vi "stat_f_s1.vi"(6 "kD":dbl=1.3, 7 "Y":dbl[](array[numeric])) -> (1 "stops":i32[](array[numeric]), 2 "starts":i32[](array[numeric]), 3 "mean":dbl format="%0.2f")   [LabVIEW 2010]
uses:
  <vilib>/Analysis/NI_AALBase.lvlib
panel:
  out "Array":i32[](array[numeric])
  out "Waveform Graph":cluster{"Numeric":i32, i32, dbl[]}(graph)
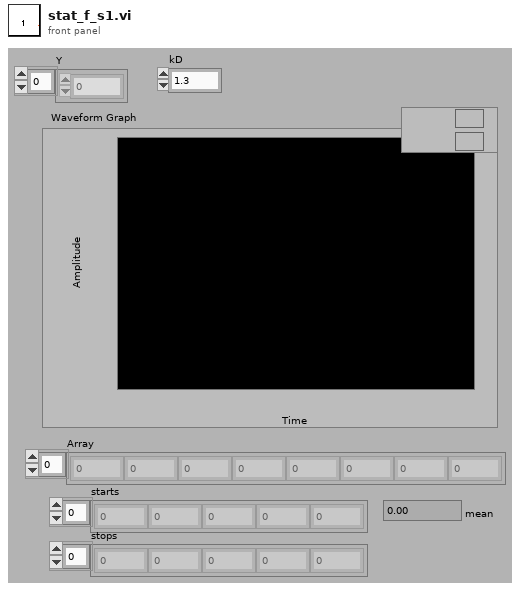
[diagram p1: front panel]
types:
  T1 = cluster{"Name":string, "Color":u32, "Style":u8, "Point Style":u8, "Name Visible":bool, "Allow Drag":bool, "Lock Style":u32, "Plot":u32, "Index":i32, "Position":cluster{"X":dbl, "Y":dbl}}[]
  T2 = cluster{"Name":string, "Color":u32, "Style":u8, "Point Style":u8, "Name Visible":bool, "Allow Drag":bool, "Lock Style":u32, "Plot":u32, "Index":i32, "Position":cluster{"X":dbl, "Y":dbl}}
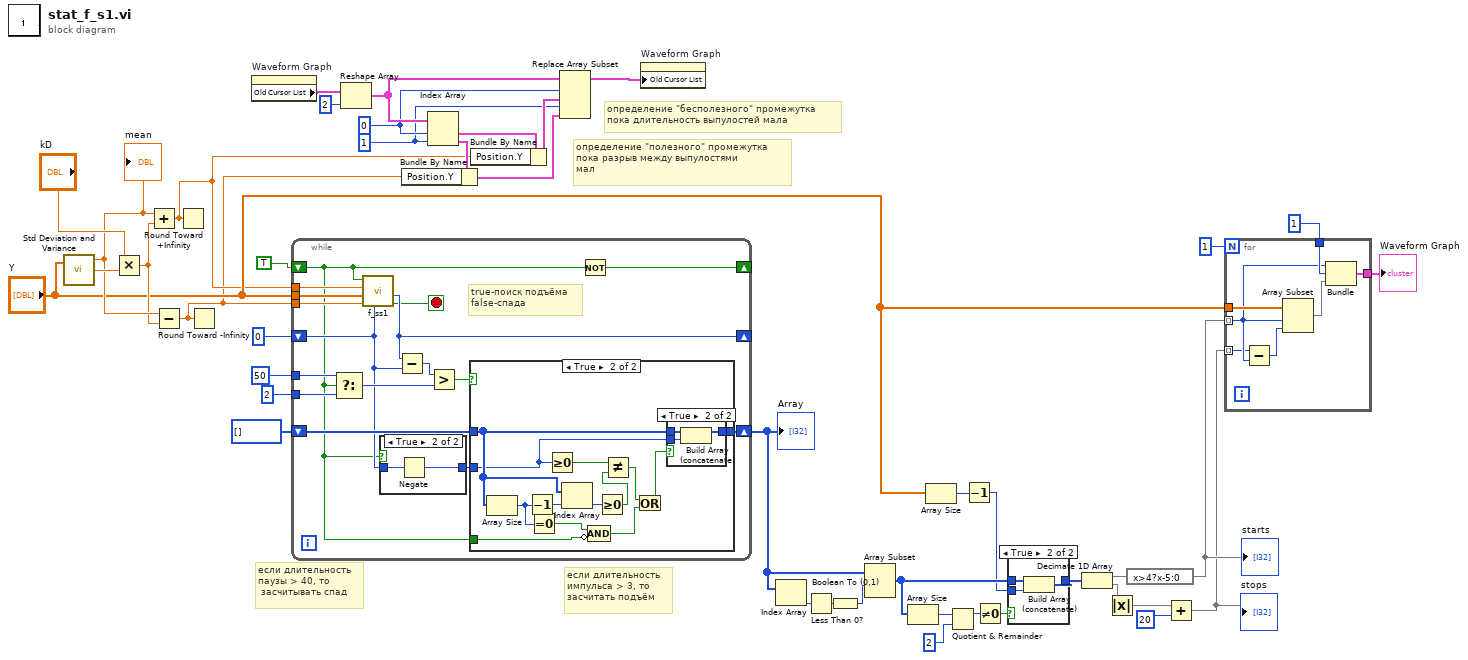
[diagram p0: block diagram]
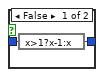
[diagram p3: hidden frame]
diagram:
  w34 = 1 ("index")
  w35 = 0 ("index")
  # "если длительность\nимпульса > 3, то\nзасчитать подъём"
  # "если длительность\nпаузы > 40, то\n засчитывать спад"
  # "определение \"полезного\" промежутка\nпока разрыв между выпулостями\nмал"
  # "определение \"бесполезного\" промежутка\nпока длительность выпулостей мала"
  n1 = call <vilib>:"Std Deviation and Variance.vi"("X"="Y") -> ("mean"=w27:dbl, "standard deviation"=w28:dbl)  [unwired: 1 in, 1 out]
  "mean" <- w27
  n2 = Multiply(x="kD", y=w28) -> (x*y=w26:dbl)
  n3 = Add(x=w27, y=w26) -> (x+y=w2:dbl)
  n4 = Subtract(x=w27, y=w26) -> (x-y=w1:dbl)
  n5 = Round Toward +Infinity(x=w2) -> ()  [unwired: 1 out]
  n6 = Round Toward -Infinity(1:w1) -> ()  [unwired: 1 out]
  n7 = property on="Waveform Graph" class="WFGraph (strict)"() -> ("Old Cursor List"=w43:T1)  [unwired: 2 in, 2 out]
  n8 = while {
    tunnel: w1 -> [w56]
    tunnel: w2 -> [w57]
    tunnel: "Y" -> [w58]
    shift-right: [w54] -> _
    shift-left: 0 -> [w46]
    shift-right: [w55] -> _
    shift-left: TRUE ("Boolean") -> [w44]
    tunnel: 50 ("t") -> [w51]
    tunnel: 2 -> [w50]
    shift-right: [w48] -> w20
    shift-left: i32[] [] -> [w47]
    stop <- w53 stop-if-true
    # "true-поиск подъёма\nfalse-спада"
    n9 = Select(t=w51, s=w44, f=w50) -> (s? t:f=w49:i32)
    n10 = call "f_ss1.vi"("index in"=w46, "lower lim"=w56, "Y"=w58, "upper lim"=w57, "Boolean"=w44) -> ("eof"=w53:bool, "index out"=w54:i32)  [unwired: 1 in, 1 out]
    n11 = case shown="True" w44 {
      tunnel: [w61 w62] -> w45
      tunnel: w46 -> [w60 w63]
      frame False {
        n12 = expression code="x>1?x-1:x"(w60) -> (w61:i32)
      }
      frame True {
        n13 = Negate(x=w63) -> (-x=w62:i32)
      }
    }
    n14 = Subtract(x=w54, y=w46) -> (x-y=w59:i32)
    n15 = Greater?(x=w59, y=w49) -> (0:w52:bool)
    n16 = case shown="True" w52 {
      tunnel: w45 -> [_ w73]
      tunnel: [w64 w77] -> w48
      tunnel: w47 -> [w64 w75]
      tunnel: w44 -> [_ w66]
      frame False {
      }
      frame True {
        n17 = Array Size(array=w75) -> (size(s)=w70:i32)
        n18 = Decrement(x=w70) -> (x-1=w76:i32)
        n19 = Equal To 0?(x=w70) -> (x = 0?=w67:bool)
        n20 = Greater Or Equal To 0?(x=w73) -> (x >= 0?=w71:bool)
        n21 = Index Array(array=w75, index=w76) -> (element=w74:i32)
        n22 = Compound Arithmetic op=AND(w67, invert w66) -> (w65:bool)
        n23 = Greater Or Equal To 0?(x=w74) -> (x >= 0?=w72:bool)
        n24 = Not Equal?(x=w71, y=w72) -> (x != y?=w69:bool)
        n25 = Or(x=w69, y=w65) -> (x .or. y?=w68:bool)
        n26 = case shown="True" w68 {
          tunnel: w73 -> [_ w81]
          tunnel: [w78 w80] -> w77
          tunnel: w75 -> [w78 w79]
          frame False {
          }
          frame True {
            n27 = Build Array (concatenate)(w79, w81) -> (w80:i32[])
          }
        }
      }
    }
    n28 = Not(x=w44) -> (.not. x?=w55:bool)
  }
  "Array" <- w20
  n29 = Reshape Array(w43, 2 ("dimension size")) -> (w39:T1)
  n30 = Index Array(array=w39, index #1=w35, index #2=w34) -> (element #1=w41:T2, element #2=w40:T2)
  n31 = Bundle By Name(cluster=w40, "Position.Y"=w1) -> (w37:T2)
  n32 = Bundle By Name(cluster=w41, "Position.Y"=w2) -> (w38:T2)
  n33 = Replace Array Subset(array=w39, new element #1=w38, index #1=w35, new element #2=w37, index #2=w34) -> (w36:T1)
  n34 = property on="Waveform Graph" class="WFGraph (strict)"("Old Cursor List"=w36) -> ()  [unwired: 2 in, 2 out]
  n35 = Index Array(array=w20) -> (element=w24:i32)  [unwired: 1 in]
  n36 = Less Than 0?(x=w24) -> (x < 0?=w23:bool)
  n37 = Boolean To (0,1)(Boolean=w23) -> (0, 1=w22:i16)
  n38 = Array Subset(array=w20, index=w22) -> (w16:i32[])  [unwired: 1 in]
  n39 = Array Size(array=w16) -> (size(s)=w15:i32)
  n40 = Array Size(array="Y") -> (size(s)=w12:i32)
  n41 = Quotient & Remainder(x=w15, y=2) -> (x-y*floor(x/y)=w18:i32)  [unwired: 1 out]
  n42 = Decrement(x=w12) -> (x-1=w14:i32)
  n43 = Not Equal To 0?(x=w18) -> (x != 0?=w17:bool)
  n44 = case shown="True" w17 {
    tunnel: w16 -> [w82 w85]
    tunnel: w14 -> [_ w84]
    tunnel: [w82 w83] -> w13
    frame False {
    }
    frame True {
      n45 = Build Array (concatenate)(w85, w84) -> (w83:i32[])
    }
  }
  n46 = Decimate 1D Array(w13) -> (w11:i32[], w21:i32[])
  n47 = Absolute Value(x=w21) -> (abs(x)=w5:i32[])
  n48 = expression code="x>4?x-5:0"(w11) -> (w6:i32[])
  "starts" <- w6
  n49 = Add(x=w5, y=20) -> (x+y=w3:i32[])
  "stops" <- w3
  n50 = for {
    N: 1 -> [_]
    tunnel: w6 -> [w88] mode=indexing
    tunnel: "Y" -> [w92]
    tunnel: w3 -> [w87] mode=indexing
    tunnel: 1 -> [w90]
    tunnel: [w89] -> w8
    n51 = Subtract(x=w87, y=w88) -> (x-y=w86:i32)
    n52 = Array Subset(array=w92, index=w88, length=w86) -> (w91:dbl[])
    n53 = Bundle("Numeric"=w88, w90, w91) -> (w89:cluster{"Numeric":i32, i32, dbl[]})  [unwired: 1 in]
  }
  "Waveform Graph" <- w8
